vi "create_wavelength_array.vi"(10 "Measurement settings":T1={"Start Wavelength (nm)"=300.0, "End Wavelength (nm)"=900.0, "Increment (nm)"=5.0, "White Bias (No. of Suns)"=1.0, "Averages per wavlength"=1.0, "Sensitivity"=17} {"Sensitivity" items=["Auto Gain"=-1, "2 nV/fA"=0, "5 nV/fA"=1, "10 nV/fA"=2, "20 nV/fA"=3, "50 nV/fA"=4, "100 nV/fA"=5, "200 nV/fA"=6, "500 nV/fA"=7, "1 uV/pA"=8, "2 uV/pA"=9, "5 uV/pA"=10, "10 uV/pA"=11, "20 uV/pA"=12, "50 uV/pA"=13, "100 uV/pA"=14, "200 uV/pA"=15, "500 uV/pA"=16, "1 mV/nA"=17, "2 mV/nA"=18, "5 mV/nA"=19, "10 mV/nA"=20, "20 mV/nA"=21, "50 mV/nA"=22, "100 mV/nA"=23, "200 mV/nA"=24, "500 mV/mA"=25, "1 V/uA"=26]; "Averages per wavlength" format="%#.2f"; "White Bias (No. of Suns)" format="%#.2f"; "End Wavelength (nm)" format="%#.2f"; "Start Wavelength (nm)" format="%#.2f"}) -> (2 "wavelengths array":dbl[](array[numeric]), 3 "number of points":i32)   [LabVIEW 2016]
uses:
  typedefs/measurement_settings.ctl
  <vilib>/Analysis/1siggen.llb/Ramp Pattern by Samples.vi
  <vilib>/Analysis/NI_AALBase.lvlib
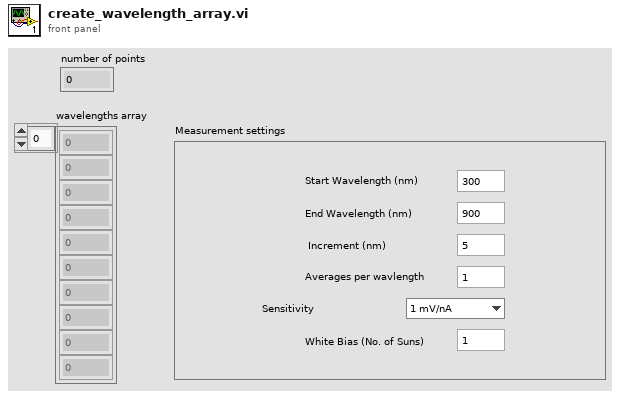
[diagram p1: front panel]
types:
  T1 = typedef "measurement_settings.ctl" = cluster{"Start Wavelength (nm)":dbl, "End Wavelength (nm)":dbl, "Increment (nm)":dbl, "White Bias (No. of Suns)":dbl, "Averages per wavlength":dbl, "Sensitivity":i16}
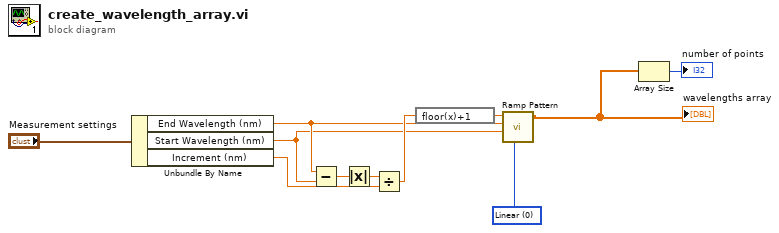
[diagram p0: block diagram]
diagram:
  w11 = u16 0 items=["Linear", "Logarithmic"] ("type")
  n1 = Unbundle By Name("Measurement settings") -> ("End Wavelength (nm)"=w6:dbl, "Start Wavelength (nm)"=w5:dbl, "Increment (nm)"=w4:dbl)
  n2 = Subtract(x=w6, y=w5) -> (x-y=w3:dbl)
  n3 = Absolute Value(x=w3) -> (abs(x)=w2:dbl)
  n4 = Divide(x=w2, y=w4) -> (x/y=w7:dbl)
  n5 = expression code="floor(x)+1"(w7) -> (w9:dbl)
  n6 = call-poly <vilib>:"Ramp Pattern.vi"("type"=w11, "start"=w5, "end"=w6, "samples"=w9) -> ("Ramp Pattern"=w8:dbl[])  [unwired: 6 in, 1 out]
  "wavelengths array" <- w8
  n7 = Array Size(array=w8) -> (size(s)=→"number of points":i32)
